vi "subOrderBuildsForTargets.vi"(6 "User Event in":T1, 8 "error in":errorcluster, 11 "Raw build order in":refnum<class "ProjectItem.lvclass">[](array[class])) -> (0 "error out":errorcluster, 3 "Build order":refnum<class "ProjectItem.lvclass">[](array[class]))   [LabVIEW 2019, in "SolutionBuilder.lvlib" / "SolutionBuilder.lvclass"]
uses:
  SolutionBuilder.lvclass
  ProjectItem/ProjectItem.lvclass
  Events/EventUpdateList.ctl
  ProjectItem/ProjectItem.lvclass/ProjectItem.ctl
  <vilib>/Utility/miscctls.llb/LVMapReplaceAction.ctl
  SolutionBuilder.lvlib
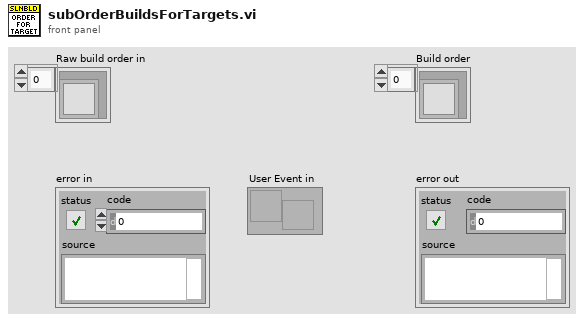
[diagram p1: front panel]
types:
  T1 = typedef "SolutionBuilder.lvlib/EventUpdateList.ctl" = refnum<user-event>
  T2 = map{string, refnum<class "ProjectItem.lvclass">[]}
  T3 = typedef "LVMapReplaceAction.ctl" = enum32{"Modify Entry only if found", "Add or Modify Entry", "Delete Entry"}
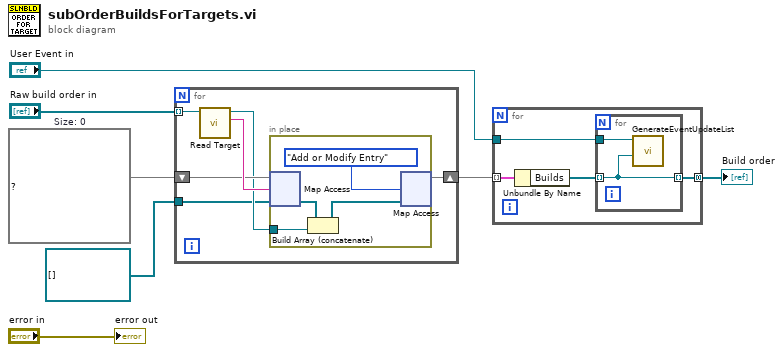
[diagram p0: block diagram]
diagram:
  w5 = T2 {}  # Size: 0
  n1 = for {
    tunnel: "Raw build order in" -> [w13] mode=indexing
    shift-right: [w11] -> w3
    shift-left: w5 -> [w10]
    tunnel: refnum<class "ProjectItem.lvclass">[] [] -> [w8]
    n2 = call "Read Target.vi"("ProjectItem in"=w13) -> ("Target"=w12:string, "ProjectItem out"=w9:refnum<class "ProjectItem.lvclass">)  [unwired: 9 in]
    n3 = in-place {
      in-place-border: w9 -> [w15]
      n4 = in-place-map #1(w10, w12, w8) -> (w17:refnum<class "ProjectItem.lvclass">[])  [unwired: 1 out]
      n5 = Build Array (concatenate)(w17, w15) -> (w14:refnum<class "ProjectItem.lvclass">[])
      n6 = in-place-map #1(w14, LVMapReplaceAction."Add or Modify Entry" ("action")) -> (w11:T2)  [unwired: 2 out]
    }
  }
  n7 = for {
    tunnel: w3 -> [w21] mode=indexing
    tunnel: [w19] -> w2 mode=concatenating
    tunnel: "User Event in" -> [w18]
    n8 = Unbundle By Name(w21) -> ("Builds"=w20:refnum<class "ProjectItem.lvclass">[])
    n9 = for {
      tunnel: w20 -> [w23] mode=indexing
      tunnel: [w23] -> w19 mode=indexing
      tunnel: w18 -> [w22]
      n10 = call "GenerateEventUpdateList.vi"("ProjectItem"=w23, "UpdateList"=w22) -> ()  [unwired: 10 in]
    }
  }
  "Build order" <- w2
  "error out" <- "error in"
